vi "monochromatorCommandGetFactor.vi"(8 "error in":errorcluster, 10 "grating":i32, 11 "monochromator":refnum<k24>) -> (0 "error out":errorcluster, 2 "factor":dbl, 3 "monochromator":refnum<k24>)   [LabVIEW 2009]
doc: "Get Factor"
uses:
  C:/Users/anderson.chen/Desktop/Software Development/Cornerstone Series API (LV9)/Cornerstone DLL/Cornerstone.dll
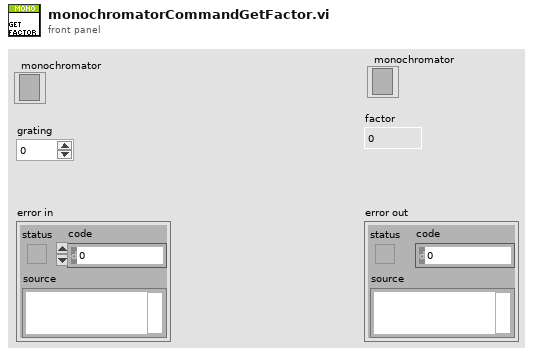
[diagram p1: front panel]
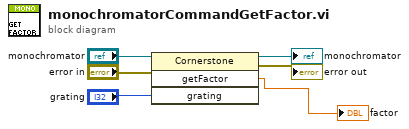
[diagram p0: block diagram]
diagram:
  n1 = invoke class="Cornerstone" method="getFactor"(reference="monochromator", error in="error in", "grating"="grating") -> (reference out=→"monochromator":refnum<k24>, error out=→"error out":errorcluster, "getFactor"=→"factor":dbl)  [unwired: 1 in, 1 out]
